vi "Configure Serial Bus (NRZ - Trigger).vi"(0 "VISA resource name":refnum<visa-resource-name>, 5 "Serial Bus Name (1: Serial Bus 1)":i32(ring)=1 items=["Serial Bus 1"=1, "Serial Bus 2"=2], 7 "Trigger Mode (0: Start Of Frame)":i32(ring) items=["Start Of Frame", "Bit Value"], 9 "Trigger Data (XXXXXXXX)":string="XXXXXXXX", 11 "error in (no error)":errorcluster, 12 "Bit Width (8)":i32=8) -> (4 "VISA resource name out":refnum<visa-resource-name>, 15 "error out":errorcluster)   [LabVIEW 2017, in "Agilent 2000 3000 X-Series.lvlib"]
doc: "Configures the trigger setting of NRZ bus.\n\n<b>Note:</b>\nThis VI is only applicable for 3000T, 4000, 6000 X-Series."
uses:
  Agilent 2000 3000 X-Series.lvlib
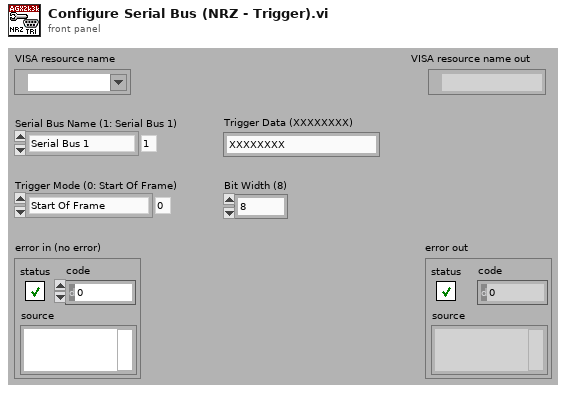
[diagram p1: front panel]
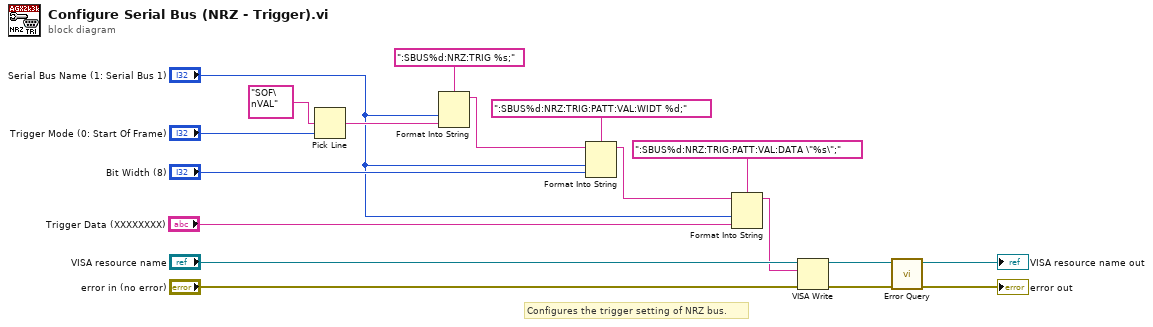
[diagram p0: block diagram]
diagram:
  # "Configures the trigger setting of NRZ bus."
  n1 = Pick Line(multi-line string="SOF\nVAL", line index="Trigger Mode (0: Start Of Frame)") -> (output string=w15:string)  [unwired: 1 in]
  n2 = Format Into String(format string=":SBUS%d:NRZ:TRIG %s;", "Serial Bus Name (1: Serial Bus 1)", w15) -> (resulting string=w4:string)  [unwired: 2 in, 1 out]
  n3 = Format Into String(format string=":SBUS%d:NRZ:TRIG:PATT:VAL:WIDT %d;", initial string=w4, "Serial Bus Name (1: Serial Bus 1)", "Bit Width (8)") -> (resulting string=w2:string)  [unwired: 1 in, 1 out]
  n4 = Format Into String(format string=":SBUS%d:NRZ:TRIG:PATT:VAL:DATA \"%s\";", initial string=w2, "Serial Bus Name (1: Serial Bus 1)", "Trigger Data (XXXXXXXX)") -> (resulting string=w3:string)  [unwired: 1 in, 1 out]
  n5 = VISA Write(VISA resource name="VISA resource name", write buffer=w3, error in (no error)="error in (no error)") -> (VISA resource name out=w8:refnum<visa-resource-name>, error out=w7:errorcluster)  [unwired: 1 out]
  n6 = call "Error Query.vi"("error in (no error)"=w7, "VISA resource name"=w8) -> ("error out"=→"error out":errorcluster, "VISA resource name out"=→"VISA resource name out":refnum<visa-resource-name>)  [unwired: 6 in, 2 out]
